vi "Arm Mode Chooser.vi"(10 "Down":bool, 11 "Up":bool) -> (3 "Down?":bool)   [LabVIEW 2011]
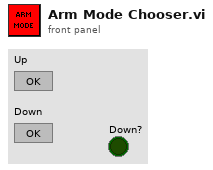
[diagram p1: front panel]
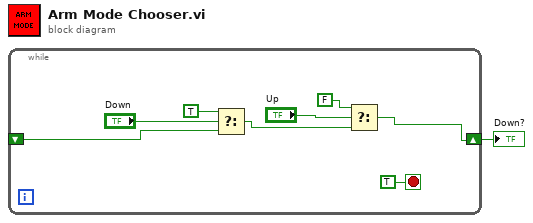
[diagram p0: block diagram]
diagram:
  n1 = while {
    shift-right: [w4] -> w1
    shift-left: _ -> [w3]
    stop <- TRUE stop-if-true
    n2 = Select(t=TRUE, s="Down", f=w3) -> (s? t:f=w2:bool)
    n3 = Select(t=FALSE, s="Up", f=w2) -> (s? t:f=w4:bool)
  }
  "Down?" <- w1
